vi "process error.vi"(10 "Error Object":refnum<class>, 11 "Template in":refnum<class "Template.lvclass">) -> ()   [LabVIEW 2020, in "Template.lvlib" / "Template.lvclass"]
doc: "Process the error acording to the definition of the application.\nThis is the last step in the error handling chain.\nIf this is the root actor, you can just call the parent method to ensure that this will close the application in case of an error."
uses:
  Template.lvclass
  C:/Program Files/National Instruments/LabVIEW 2020/vi.lib/ActorFramework/Actor/Actor.lvclass
  <vilib>/ActorFramework/Actor/Actor.lvclass/Actor.ctl
  <vilib>/ActorFramework/Message Enqueuer/Message Enqueuer.lvclass/Message Enqueuer.ctl
  <vilib>/ActorFramework/Stop Msg/Stop Msg.lvclass/Stop Msg.ctl
  <vilib>/ActorFramework/Message Enqueuer/Enqueue Critical.vi
  <vilib>/ActorFramework/Message Enqueuer/Init from Existing Queue.vi
  <vilib>/ActorFramework/Stop Msg/Stop Msg.lvclass
  C:/Program Files/National Instruments/LabVIEW 2020/vi.lib/ActorFramework/Message/Message.lvclass
  <vilib>/ActorFramework/Message Priority Queue/Priority Enqueue.vi
  <vilib>/ActorFramework/Message Enqueuer/Message Enqueuer.lvclass
  interfaces/Error Interface/Error/Error.lvclass
  <vilib>/ActorFramework/Actor/Actor.lvclass
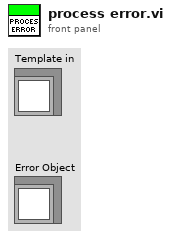
[diagram p1: front panel]
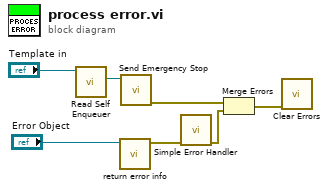
[diagram p0: block diagram]
diagram:
  n1 = call <vilib>:"Read Self Enqueuer.vi"("Actor"="Template in") -> ("Self Enqueuer"=w2:refnum<class "Message Enqueuer.lvclass">)  [unwired: 10 in]
  n2 = call "return error info.vi"("Error in"="Error Object") -> ("Error to Process"=w6:errorcluster)  [unwired: 7 in, 3 out]
  n3 = call <vilib>:"Send Emergency Stop.vi"("Message Enqueuer"=w2) -> ("error out"=w7:errorcluster)  [unwired: 10 in]
  n4 = call <vilib>:"Simple Error Handler.vi"("error in (no error)"=w6) -> ("error out"=w5:errorcluster)  [unwired: 4 in, 4 out]
  n5 = Merge Errors(w7, w5) -> (w1:errorcluster)
  n6 = call <vilib>:"Clear Errors.vi"("error in (no error)"=w1) -> ()  [unwired: 5 in, 2 out]
